vi "Write_queue_data.vi"(0 "Queue DVR in":refnum<data-value>, 5 "DATA":T1, 11 "error in (no error)":errorcluster) -> (4 "Queue DVR out":refnum<data-value>, 15 "error out":errorcluster)   [LabVIEW 2020, in "Data Communication Transmitter.lvlib" / "Queue.lvclass"]
uses:
  Classes/Children/Intra-Application/Children/With Data/Children/Queues/Queue.lvclass
  Classes/Children/Intra-Application/Children/With Data/Children/Queues/Queue.lvclass/Queue.ctl
  Accessors/Write/Write DATA.vi
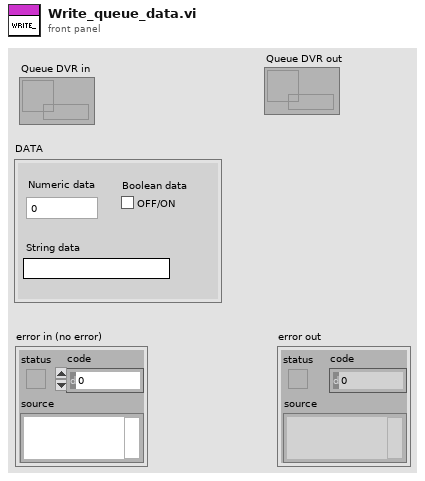
[diagram p1: front panel]
types:
  T1 = cluster{"Numeric data":dbl, "String data":string, "Boolean data":bool}
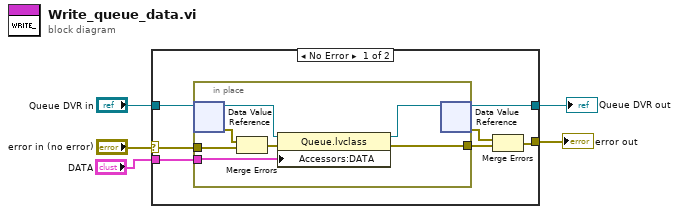
[diagram p0: block diagram]
diagram:
  n1 = case shown="No Error" "error in (no error)" {
    selector: "error in (no error)" -> [w11 w21]
    tunnel: [w8 w21] -> w4
    tunnel: "Queue DVR in" -> [w12 w20]
    tunnel: [w7 w20] -> w2
    tunnel: "DATA" -> [w6 _]
    frame No Error {
      n2 = in-place "In Place Element Structure" {
        in-place-border: [w16] -> w10
        in-place-border: w11 -> [w19]
        in-place-border: w6 -> [w13]
        n3 = in-place-dvr #1(w12) -> (w15:refnum<class "Queue.lvclass">, w18:errorcluster)
        n4 = Merge Errors(w18, w19) -> (w17:errorcluster)
        n5 = property on="Property Node" class="Queue.lvclass"(reference=w15, error in=w17, "Accessors:DATA"=w13) -> (reference out=w14:refnum<class "Queue.lvclass">, error out=w16:errorcluster)
        n6 = in-place-dvr #1(w14) -> (w7:refnum<data-value>, w9:errorcluster)
      }
      n7 = Merge Errors(w9, w10) -> (w8:errorcluster)
    }
    frame Error {
    }
  }
  "error out" <- w4
  "Queue DVR out" <- w2
